vi "oax_Set Waveform Chart Property.vi"(5 "reset? (T)":bool=TRUE, 8 "error in (no error)":errorcluster, 9 "channel color":u32[](array[numeric]), 10 "channel name":string[](array[string]), 11 "Waveform Chart ref":refnum<vi>) -> (0 "error out":errorcluster)   [LabVIEW 2017]
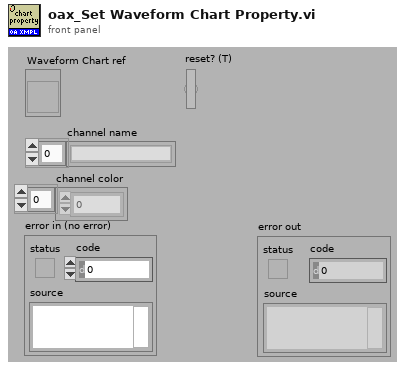
[diagram p1: front panel]
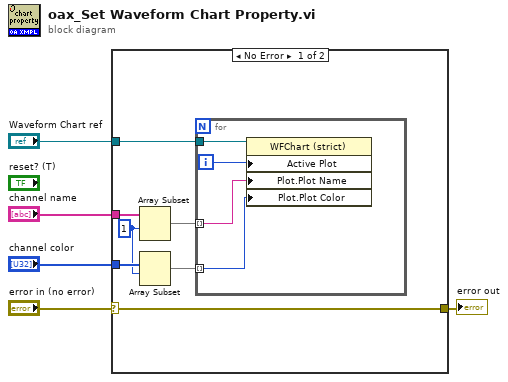
[diagram p0: block diagram]
diagram:
  n1 = case shown="No Error" "error in (no error)" {
    selector: "error in (no error)" -> [w6 w17]
    tunnel: [w6 w17] -> w4
    tunnel: "Waveform Chart ref" -> [w12 _]
    tunnel: "channel name" -> [w11 _]
    tunnel: "channel color" -> [w10 _]
    frame No Error {
      w9 = 1 ("index")
      n2 = Array Subset(array=w11, index=w9) -> (w8:string[])  [unwired: 1 in]
      n3 = Array Subset(array=w10, index=w9) -> (w7:u32[])  [unwired: 1 in]
      n4 = for {
        tunnel: w12 -> [w16]
        tunnel: w8 -> [w14] mode=indexing
        tunnel: w7 -> [w13] mode=indexing
        i -> [w15]
        n5 = property class="WFChart (strict)"(reference=w16, "Active Plot"=w15, "Plot.Plot Name"=w14, "Plot.Plot Color"=w13) -> ()  [unwired: 1 in, 2 out]
      }
    }
    frame Error {
    }
  }
  "error out" <- w4
